vi "getTCPSendPath.vi"(1 "Data cluster out":T1) -> (0 "Path":path)   [LabVIEW 2009]
uses:
  dataCluster.ctl
  <vilib>/vision/Image Controls.llb/IMAQ Image.ctl
  DataQueueTypeDef.ctl
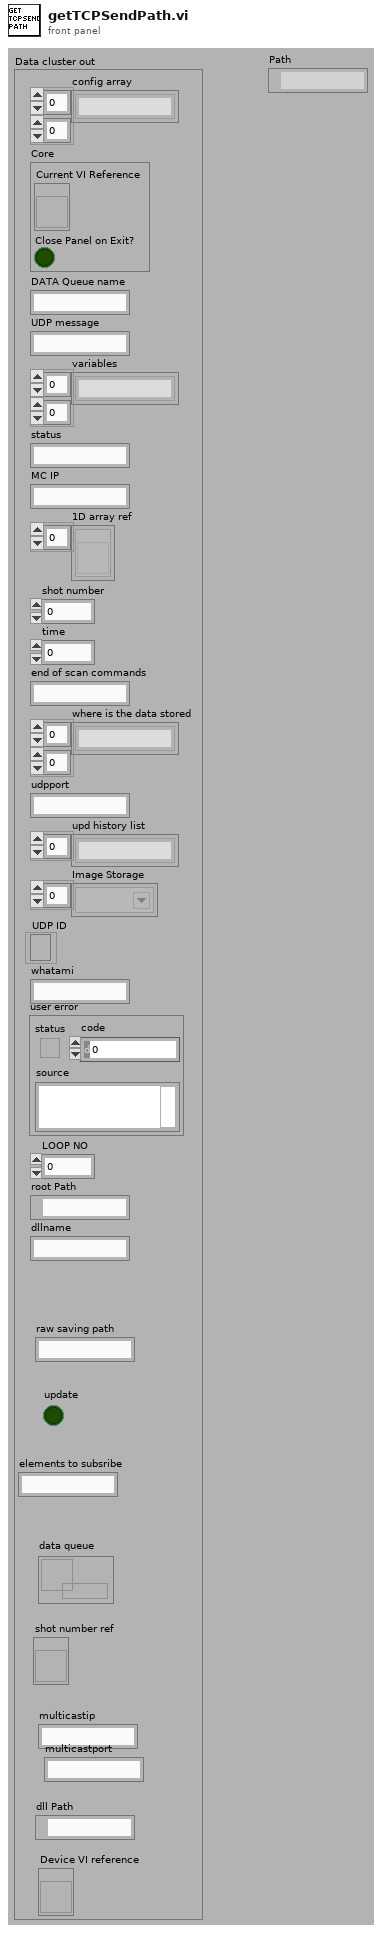
[diagram p1: front panel]
types:
  T1 = typedef "dataCluster.ctl" = cluster{"config array":string[][], "Core":cluster{"Current VI Reference":refnum<vi>, "Close Panel on Exit?":bool}, "DATA Queue name":string, "UDP message":string, "variables":string[][], "status":string, "MC IP":string, "1D array ref":refnum<vi>[], "shot number":i32, "time":u32, "end of scan commands":string, "where is the data stored":string[][], "udpport":string, "upd history list":string[], "Image Storage":T2[], "UDP ID":refnum<k16>, "whatami":string, "user error":errorcluster, "LOOP NO":u32, "root Path":path, "dllname":string, "raw saving path":string, "update":bool, "elements to subsribe":string, "data queue":refnum<queue>, "shot number ref":refnum<vi>, "multicastip":string, "multicastport":string, "dll Path":path, "Device VI reference":refnum<vi>}
  T2 = typedef "IMAQ Image.ctl" = refnum<image>
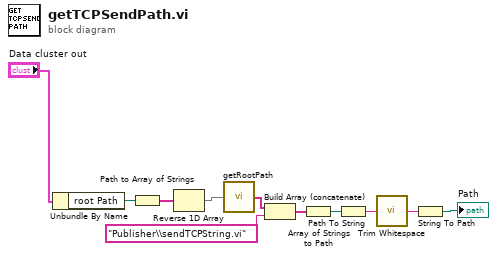
[diagram p0: block diagram]
diagram:
  n1 = Unbundle By Name("Data cluster out") -> ("root Path"=w1:path)
  n2 = Path to Array of Strings(0:w1) -> (2:w3:string[])  [unwired: 1 out]
  n3 = Reverse 1D Array(array=w3) -> (reversed array=w4:string[])
  n4 = call "getRootPath.vi"("Array 2"=w4) -> ("Array"=w10:string[])
  n5 = Build Array (concatenate)(w10, "Publisher\\sendTCPString.vi") -> (w8:string[])
  n6 = Array of Strings to Path(0:w8) -> (2:w7:path)  [unwired: 1 in]
  n7 = Path To String(path=w7) -> (string=w6:string)
  n8 = call <vilib>:"Trim Whitespace.vi"("string"=w6) -> ("trimmed string"=w5:string)  [unwired: 1 in]
  n9 = String To Path(string=w5) -> (path=→"Path":path)
